vi "Set Source Value.vi"(8 "error in (no error)":errorcluster, 9 "Source Value Units":T1, 10 "Source Value":dbl, 11 "Stanford Research PS350 in":refnum<class "Stanford Research PS350.lvclass">) -> (0 "error out":errorcluster, 3 "Stanford Research PS350 out":refnum<class "Stanford Research PS350.lvclass">)   [LabVIEW 2011, in "Stanford Research PS350.lvclass"]
uses:
  Stanford Research PS350.lvclass
  Power Supply/Source Units.ctl
  Stanford Research PS350.lvclass/Stanford Research PS350.ctl
  3rd Party/Stanford Research PS300 Series/Stanford Research PS300 Series.lvlib
  Power Supply/Power Supply.lvclass
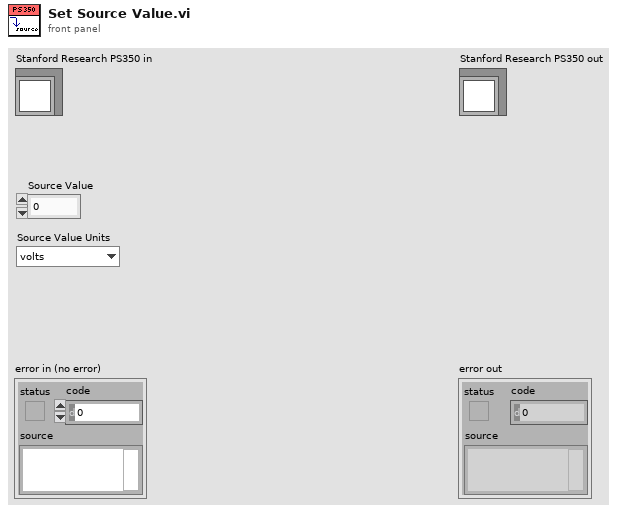
[diagram p1: front panel]
types:
  T1 = typedef "Power Supply.lvclass/Source Units.ctl" = enum16{"volts", "millivolts", "microvolts", "amps", "milliamps", "microamps", "nanoamps"}
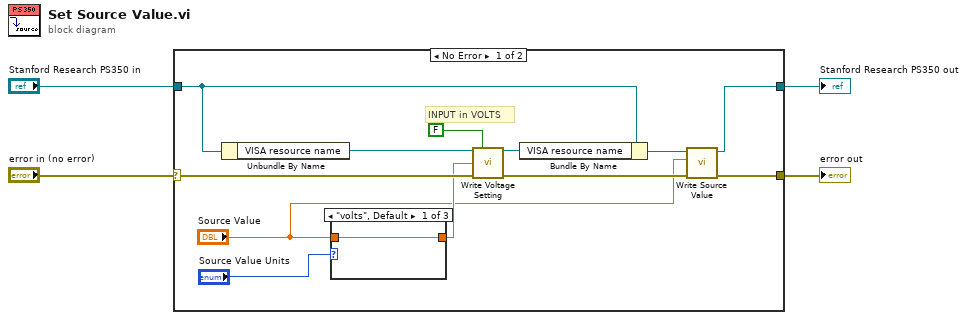
[diagram p0: block diagram]
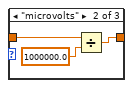
[diagram p2: hidden frame]
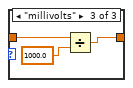
[diagram p3: hidden frame]
diagram:
  n1 = case shown="No Error" "error in (no error)" {
    selector: "error in (no error)" -> [w15 w25]
    tunnel: [w7 w25] -> w3
    tunnel: [w6 w24] -> w1
    tunnel: "Stanford Research PS350 in" -> [w13 w24]
    frame No Error {
      # "INPUT in VOLTS"
      n2 = Unbundle By Name(w13) -> ("VISA resource name"=w14:refnum<visa-resource-name>)
      n3 = case shown="\"volts\", Default" "Source Value Units" {
        tunnel: "Source Value" -> [w17 w19 w22]
        tunnel: [w17 w18 w23] -> w10
        frame "volts", Default {
        }
        frame "microvolts" {
          n4 = Divide(x=w19, y=1000000.0) -> (x/y=w18:dbl)
        }
        frame "millivolts" {
          n5 = Divide(x=w22, y=1000.0) -> (x/y=w23:dbl)
        }
      }
      n6 = call "Write Voltage Setting.vi"("VISA resource name"=w14, "Enable Voltage Inversion (T: Enabled)"=FALSE, "Voltage Setting (100.00)"=w10, "error in (no error)"=w15) -> ("VISA resource name out"=w12:refnum<visa-resource-name>, "error out"=w9:errorcluster)  [unwired: 10 in]
      n7 = Bundle By Name(cluster=w13, "VISA resource name"=w12) -> (w8:refnum<class "Stanford Research PS350.lvclass">)
      n8 = call-dynamic "Write Source Value.vi"("error in (no error)"=w9, "Source Value"="Source Value", "Power Supply in"=w8) -> ("error out"=w7:errorcluster, "Power Supply out"=w6:refnum<class "Stanford Research PS350.lvclass">)  [unwired: 7 in]
    }
    frame Error {
    }
  }
  "error out" <- w3
  "Stanford Research PS350 out" <- w1
